vi "Read Position.vi"(8 "error in (no error)":errorcluster, 10 "No. of attempts (3)":i32=3, 11 "Scientifica XYZ Gen1 in":refnum<class "Scientifica XYZ Gen1.lvclass">) -> (0 "error out":errorcluster, 1 "No Feedback":bool, 2 "XYZ Coordinates":T1 {"Z" format="Z= %#_g"; "Y" format="Y= %#_g"; "X" format="X= %#_g"}, 3 "Scientifica XYZ Gen1 out":refnum<class "Scientifica XYZ Gen1.lvclass">)   [LabVIEW 2020, in "TranslationStageClassStructure.lvlib" / "Scientifica XYZ Gen1.lvclass"]
uses:
  Scientifica XYZ Gen1.lvclass
  Typedefs/XYZ_coordinates.ctl
  Scientifica XYZ Gen1.lvclass/Scientifica XYZ Gen1.ctl
  Serial Comms/Serial Comms/Serial Comms.lvclass
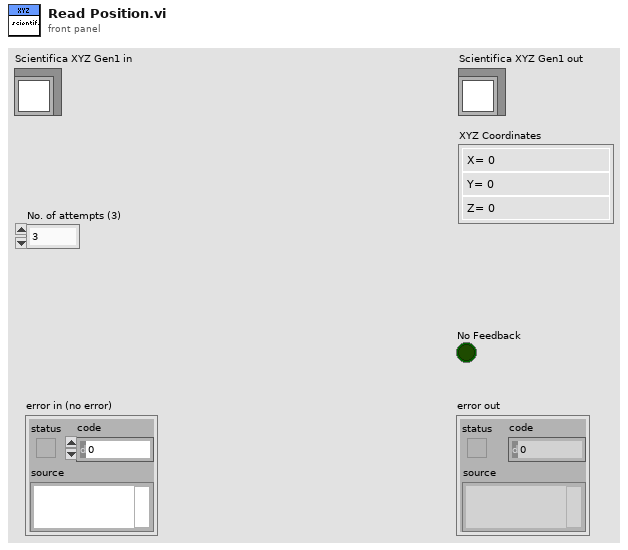
[diagram p1: front panel]
types:
  T1 = typedef "XYZ_coordinates.ctl" = cluster{"X":sgl, "Y":sgl, "Z":sgl}
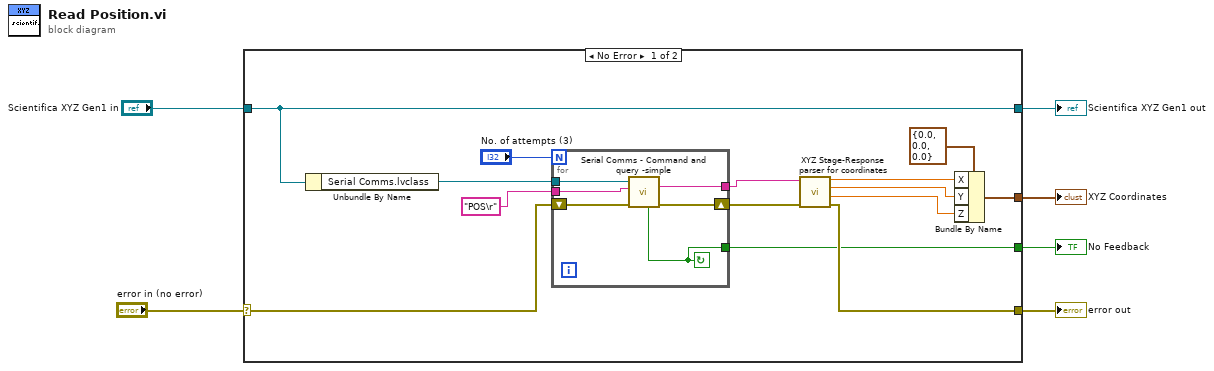
[diagram p0: block diagram]
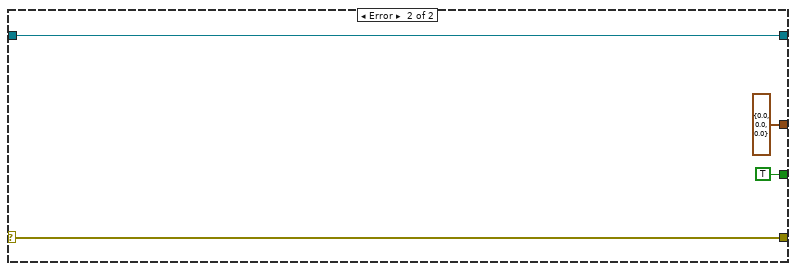
[diagram p2: hidden frame]
diagram:
  n1 = case shown="No Error" "error in (no error)" {
    selector: "error in (no error)" -> [w18 w30]
    tunnel: [w10 w30] -> w5
    tunnel: [w20 w29] -> w3
    tunnel: "Scientifica XYZ Gen1 in" -> [w20 w29]
    tunnel: [w9 cluster{"X":sgl, "Y":sgl, "Z":sgl} {"X"=0.0, "Y"=0.0, "Z"=0.0} ("Stage XYZ Position")] -> w2
    tunnel: [w7 TRUE ("Empty response string")] -> w1
    frame No Error {
      n2 = Unbundle By Name(w20) -> ("Serial Comms.lvclass"=w19:refnum<class "Serial Comms.lvclass">)
      n3 = for {
        N: "No. of attempts (3)" -> [_]
        tunnel: w19 -> [w26]
        shift-right: [w24] -> w12
        shift-left: w18 -> [w25]
        tunnel: "POS\r" ("string to write") -> [w23]
        tunnel: [w22] -> w11
        tunnel: [w21] -> w7
        stop <- w21 continue-if-true
        n4 = call "Serial Comms - Command and query -simple.vi"("error in (no error)"=w25, "string to write"=w23, "Serial Comms in"=w26) -> ("error out"=w24:errorcluster, "read string"=w22:string, "Empty response string"=w21:bool)  [unwired: 4 in, 2 out]
      }
      n5 = call "XYZ Stage-Response parser for coordinates.vi"("error in (no error)"=w12, "Filtered response string (no CR)"=w11) -> ("error out"=w10:errorcluster, "Z"=w15:sgl, "Y"=w14:sgl, "X"=w13:sgl)  [unwired: 6 in]
      n6 = Bundle By Name(cluster=T1 {"X"=0.0, "Y"=0.0, "Z"=0.0} ("XYZ Coordinates"), "X"=w13, "Y"=w14, "Z"=w15) -> (w9:T1)
    }
    frame Error {
    }
  }
  "error out" <- w5
  "Scientifica XYZ Gen1 out" <- w3
  "No Feedback" <- w1
  "XYZ Coordinates" <- w2
